vi "Read File Location.vi"(8 "error in (no error)":errorcluster, 11 "UserPreferencesFileManager in":refnum<class "User Preferences File.lvclass">) -> (0 "error out":errorcluster, 2 "File Location":path, 3 "UserPreferencesFileManager out":refnum<class "User Preferences File.lvclass">)   [LabVIEW 2020, in "RxnRover.lvlib" / "User Preferences File.lvclass"]
uses:
  User Preferences File.lvclass
  User Preferences File.lvclass/User Preferences File.ctl
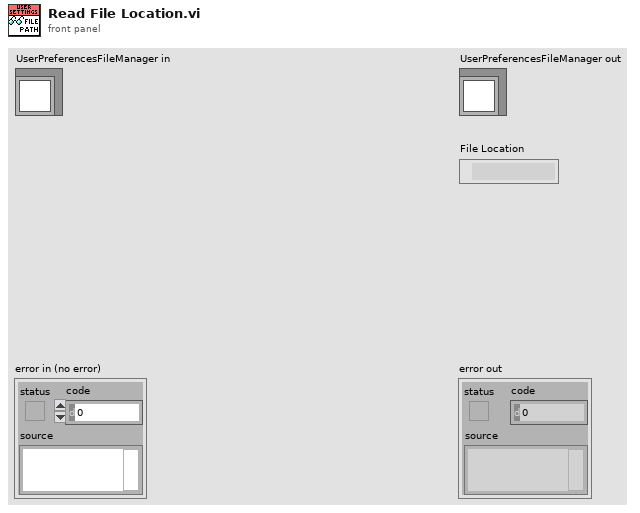
[diagram p1: front panel]
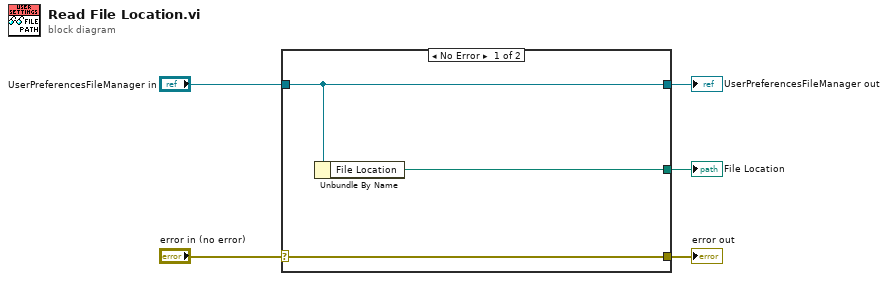
[diagram p0: block diagram]
diagram:
  n1 = case shown="No Error" "error in (no error)" {
    selector: "error in (no error)" -> [w8 w9]
    tunnel: [w8 w9] -> w4
    tunnel: [w7 w10] -> w2
    tunnel: "UserPreferencesFileManager in" -> [w7 w10]
    tunnel: [w6 _] -> w1
    frame No Error {
      n2 = Unbundle By Name(w7) -> ("File Location"=w6:path)
    }
    frame Error {
    }
  }
  "error out" <- w4
  "UserPreferencesFileManager out" <- w2
  "File Location" <- w1
